vi "Update Listbox.vi"(8 "error in (no error)":errorcluster, 10 "ListBox in":refnum<vi>, 11 "Node Ptr":T1 format="%.0x") -> (0 "error out":errorcluster, 3 "Item Ref out":T1 format="%.0x")   [LabVIEW 2016, in "FPGA Addon System Explorer.lvlib"]
uses:
  FPGA Addon System Explorer.lvlib
  <vilib>/NI Veristand/Custom Device API/Custom Device Item Ref.ctl
  FPGA resource mapping.ctl
  FPGA-Resource-Manager-APIs/Source/Channel Type.ctl
  <vilib>/NI Veristand/Custom Device API/Get Item Property (Variant).vi
  FPGA-Resource-Manager-APIs/Source/System Definition/FPGA RM System Definition API.lvlib
  <vilib>/NI VeriStand/Custom Device API/Custom Device API.lvlib
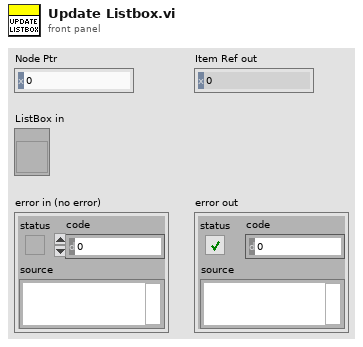
[diagram p1: front panel]
types:
  T1 = typedef "Custom Device API.lvlib/Custom Device Item Ref.ctl" = u64
  T2 = typedef "FPGA RM System Definition API.lvlib/FPGA resource mapping.ctl" = cluster{"name":string, "datatype":variant, "channel type":T3}
  T3 = typedef "FPGA RM System Definition API.lvlib/Channel Type.ctl" = enum16{"Write Channel", "Read Channel", "Write Waveform", "Read Waveform"}
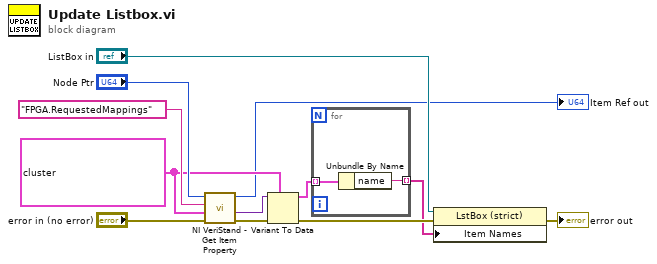
[diagram p0: block diagram]
diagram:
  w3 = T2[] [{"name"="", "datatype"=variant, "channel type"=enum."Write Channel"}] ("Array")
  n1 = call-poly <vilib>:"NI VeriStand - Get Item Property.vi"("error in (no error)"="error in (no error)", "Default Value"=w3, "Property Name"="FPGA.RequestedMappings", "Item Ref in"="Node Ptr") -> ("error out"=w5:errorcluster, "Value"=w4:variant, "Item Ref out"=→"Item Ref out":T1)  [unwired: 4 in, 1 out]
  n2 = Variant To Data(error in=w5, type=w3, Variant=w4) -> (data=w8:T2[], error out=w11:errorcluster)
  n3 = for {
    tunnel: w8 -> [w14] mode=indexing
    tunnel: [w13] -> w9 mode=indexing
    n4 = Unbundle By Name(w14) -> ("name"=w13:string)
  }
  n5 = property on="Property Node" class="LstBox (strict)"(reference="ListBox in", error in=w11, "Item Names"=w9) -> (error out=→"error out":errorcluster)  [unwired: 1 out]
